vi "Send Shutdown Command.vi"(8 "error in (no error)":errorcluster, 11 "Plugin Interface in":refnum<class "Plugin Interface.lvclass">) -> (0 "error out":errorcluster, 3 "Plugin Interface out":refnum<class "Plugin Interface.lvclass">)   [LabVIEW 2017, in "DSF Core.lvlib" / "Plugin Interface.lvclass"]
uses:
  Interface/Plugin/Plugin Interface.lvclass
  C:/Git/DSF/Core/Classes/Interface/Interface.lvclass
  Interface/Plugin/Command Data.ctl
  Interface/Plugin/Command.ctl
  Interface/Plugin/Command Parameters.ctl
  Interface/Plugin/Response.ctl
  Interface/Plugin/Send Plugin Command.vi
  Interface/Plugin/Wait For Plugin Response.vi
  Interface/Dispatcher/Invalid Response.vi
  Interface/Interface.lvclass
  DSF Core.lvlib
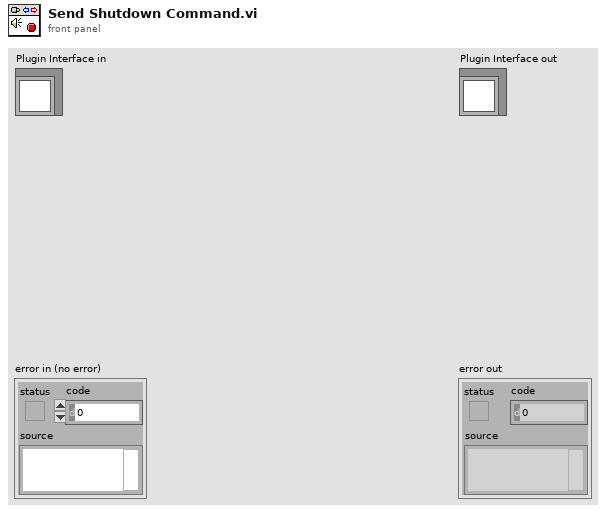
[diagram p1: front panel]
types:
  T1 = typedef "DSF Core.lvlib/Plugin Interface.lvclass/Command Data.ctl" = cluster{"Command":T2, "Parameters":T3}
  T2 = typedef "DSF Core.lvlib/Plugin Interface.lvclass/Command.ctl" = enum8{"Idle", "Start", "Set Inline Buffer", "Rx", "Tx", "Shutdown"}
  T3 = typedef "DSF Core.lvlib/Plugin Interface.lvclass/Command Parameters.ctl" = cluster{"arg1":u64, "arg2":u64}
  T4 = typedef "DSF Core.lvlib/Plugin Interface.lvclass/Response.ctl" = enum8{"General Ack", "Shutting Down"}
  T5 = typedef "DSF Core.lvlib/Plugin Interface.lvclass/Response Data.ctl" = cluster{"Response":T4, "Parameters":T6}
  T6 = typedef "DSF Core.lvlib/Plugin Interface.lvclass/Response Parameters.ctl" = cluster{"arg1":u64, "arg2":u64}
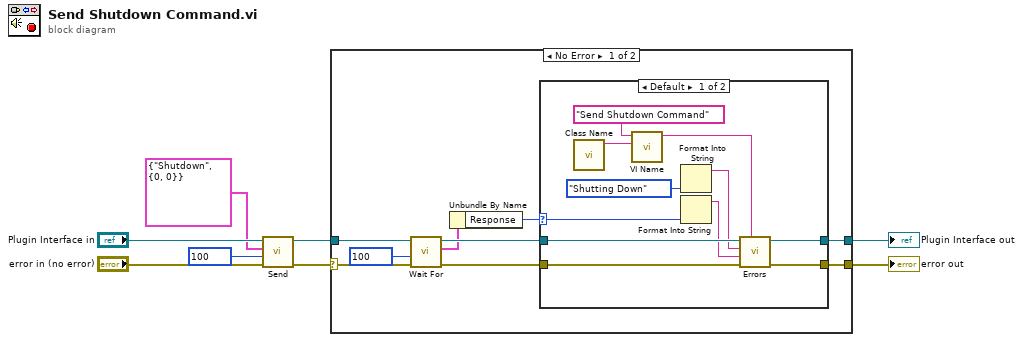
[diagram p0: block diagram]
diagram:
  n1 = call-poly "Send.vi"("error in (no error)"="error in (no error)", "timeout in ms (0)"=100, "command"=T1 {"Command"=enum."Shutdown", "Parameters"={"arg1"=0, "arg2"=0}}, "Plugin Interface in"="Plugin Interface in") -> ("error out"=w4:errorcluster, "Plugin Interface out"=w5:refnum<class "Plugin Interface.lvclass">)  [unwired: 6 in]
  n2 = case shown="No Error" w4 {
    selector: w4 -> [w11 w31]
    tunnel: w5 -> [w14 w32]
    tunnel: [w17 w31] -> w8
    tunnel: [w16 w32] -> w7
    frame No Error {
      n3 = call-poly "Wait For.vi"("error in (no error)"=w11, "timeout in ms (0)"=100, "Plugin Interface in"=w14) -> ("error out"=w12:errorcluster, "response"=w9:T5, "Plugin Interface out"=w13:refnum<class "Plugin Interface.lvclass">)  [unwired: 5 in, 1 out]
      n4 = Unbundle By Name(w9) -> ("Response"=w15:T4)
      n5 = case shown="Default" w15 {
        selector: w15 -> [w22 _]
        tunnel: w12 -> [w27 w30]
        tunnel: [w25 w30] -> w17
        tunnel: w13 -> [w28 w29]
        tunnel: [w26 w29] -> w16
        frame Default {
          n6 = call "Class Name.vi"() -> ("class name"=w20:string)  [unwired: 11 in]
          n7 = call "VI Name.vi"("class name (\"\")"=w20, "vi name"="Send Shutdown Command" ("error source vi name")) -> ("full VI name"=w18:string)  [unwired: 9 in]
          n8 = Format Into String(Response."Shutting Down" ("x")) -> (resulting string=w23:string)  [unwired: 3 in, 1 out]
          n9 = Format Into String(w22) -> (resulting string=w21:string)  [unwired: 3 in, 1 out]
          n10 = call-poly "Errors.vi"("error source vi name"=w18, "error in (no error)"=w27, "actual response"=w21, "expected response"=w23, "Interface in"=w28) -> ("error out"=w25:errorcluster, "Interface out"=w26:refnum<class "Plugin Interface.lvclass">)  [unwired: 5 in]
        }
        frame "Shutting Down" {
        }
      }
    }
    frame Error {
    }
  }
  "error out" <- w8
  "Plugin Interface out" <- w7
